vi "FMDLConfigKeithley2450TriggerModelForAmmeterDataToUserBufferWithMultipleReadings.vi"(2 "Trigger Count (1)":i32=1 format="%#.6g", 3 "error in (no error)":errorcluster, 4 "Buffer Name (defbuffer1)":string="defbuffer1", 5 "VISA resource name":refnum<visa-resource-name>) -> (0 "error out":errorcluster, 1 "VISA resource name out":refnum<visa-resource-name>)   [LabVIEW 2018]
uses:
  <instrlib>/Keithley 2450/Keithley 2450.lvlib
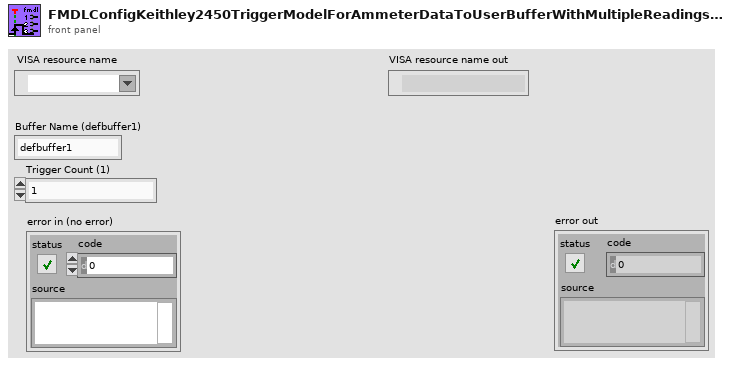
[diagram p1: front panel]
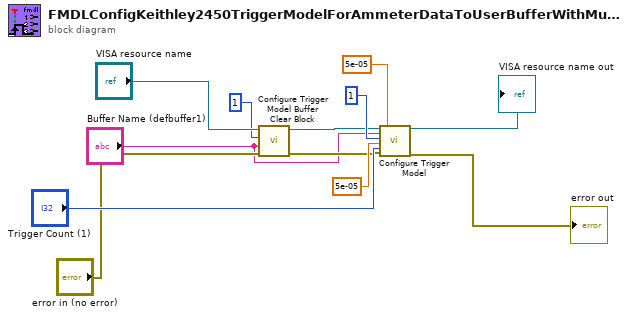
[diagram p0: block diagram]
diagram:
  n1 = call <instrlib>:"Configure Trigger Model Buffer Clear Block.vi"("error in (no error)"="error in (no error)", "Buffer Name (defbuffer1)"="Buffer Name (defbuffer1)", "Block Number (1)"=1, "VISA resource name"="VISA resource name") -> ("error out"=w5:errorcluster, "VISA resource name out"=w3:refnum<visa-resource-name>)  [unwired: 6 in]
  n2 = call <instrlib>:"Configure Trigger Model.vi"("VISA resource name"=w3, "Buffer Name (defbuffer1)"="Buffer Name (defbuffer1)", "Number of Times to repeat (1)"=1, "Timer Interval (1us)"=5e-05, "Trigger Count (1)"="Trigger Count (1)", "error in (no error)"=w5, "Trigger Delay (1 us)"=5e-05) -> ("VISA resource name out"=→"VISA resource name out":refnum<visa-resource-name>, "error out"=→"error out":errorcluster)  [unwired: 11 in]
